vi "Работа с бинарным файлом knob.vi"() -> ()   [LabVIEW 2021]
panel:
  out "data":dbl[](array[numeric])
  out "XY Graph":cluster{i32[], dbl[]}(graph)
  out "Waveform Chart":dbl[](graph)
  in  "Knob":dbl(knob) scale=0.0..10.0
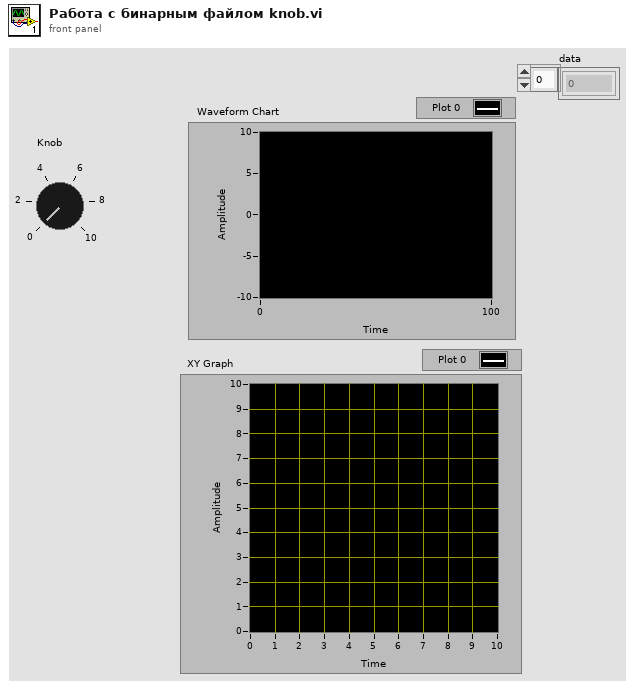
[diagram p1: front panel]
types:
  T1 = enum16{"open", "replace", "create", "open or create", "replace or create", "replace or create with confirmation"}
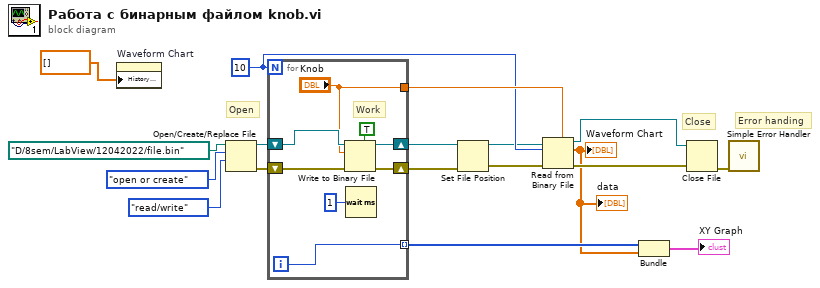
[diagram p0: block diagram]
diagram:
  w9 = 10
  # "Error handing"
  # "Close"
  # "Open"
  n1 = property on="Waveform Chart" class="WFChart (strict)"("History Data"=dbl[] []) -> ()  [unwired: 2 in, 2 out]
  n2 = Open/Create/Replace File(file path (use dialog)=path "D:/8sem/LabView/12042022/file.bin", operation (0:open)=T1."open or create", access (0:read/write)=enum16{"read/write", "read-only", "write-only"}."read/write") -> (refnum out=w14:refnum<file>, error out=w15:errorcluster)  [unwired: 3 in, 1 out]
  n3 = for {
    N: w9 -> [_]
    shift-right: [w25] -> w4
    shift-left: w15 -> [w26]
    shift-right: [w24] -> w7
    shift-left: w14 -> [w23]
    tunnel: ["Knob"] -> w10
    tunnel: [w19] -> w3 mode=indexing
    i -> [w19]
    # "Work"
    n4 = Write to Binary File(file (use dialog)=w23, data="Knob", error in=w26, 5:TRUE ("prepend array or string size? (T)")) -> (refnum out=w24:refnum<file>, error out=w25:errorcluster)  [unwired: 2 in, 1 out]
    n5 = Wait (ms)(milliseconds to wait=u32 1) -> ()  [unwired: 1 out]
  }
  n6 = Set File Position(refnum=w7, error in=w4) -> (refnum out=w6:refnum<file>, error out=w5:errorcluster)  [unwired: 2 in]
  n7 = Read from Binary File(5:w10, 8:w5, 10:w9, 11:w6) -> (0:w12:errorcluster, 2:w2:dbl[], 3:w11:refnum<file>)  [unwired: 2 in, 1 out]
  "Waveform Chart" <- w2
  "data" <- w2
  n8 = Bundle(w3, w2) -> (→"XY Graph":cluster{i32[], dbl[]})  [unwired: 1 in]
  n9 = Close File(refnum=w11, error in=w12) -> (error out=w16:errorcluster)  [unwired: 1 out]
  n10 = call <vilib>:"Simple Error Handler.vi"("error in (no error)"=w16) -> ()  [unwired: 4 in, 5 out]
